vi "Matrix_Create.vi"(9 "Columns":i32, 11 "Rows":i32) -> (3 "output matrix":T1)   [LabVIEW 2019, in "Trajectory_Library.lvlib"]
doc: "Constructs an empty zero matrix of the given dimensions. \n\nInputs:\n - rows -- The number of rows of the matrix.\n - columns -- The number of columns of the matrix.\n\nOutputs:\n - output matrix -- Newly created matrix"
uses:
  Trajectory_Library.lvlib
  <vilib>/Analysis/Matrix/Datatypes/RealMatrix.ctl
  <vilib>/Analysis/Matrix/NI_Matrix.lvlib
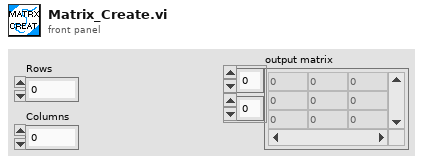
[diagram p1: front panel]
types:
  T1 = typedef "NI_Matrix.lvlib/RealMatrix.ctl" = dbl[][]
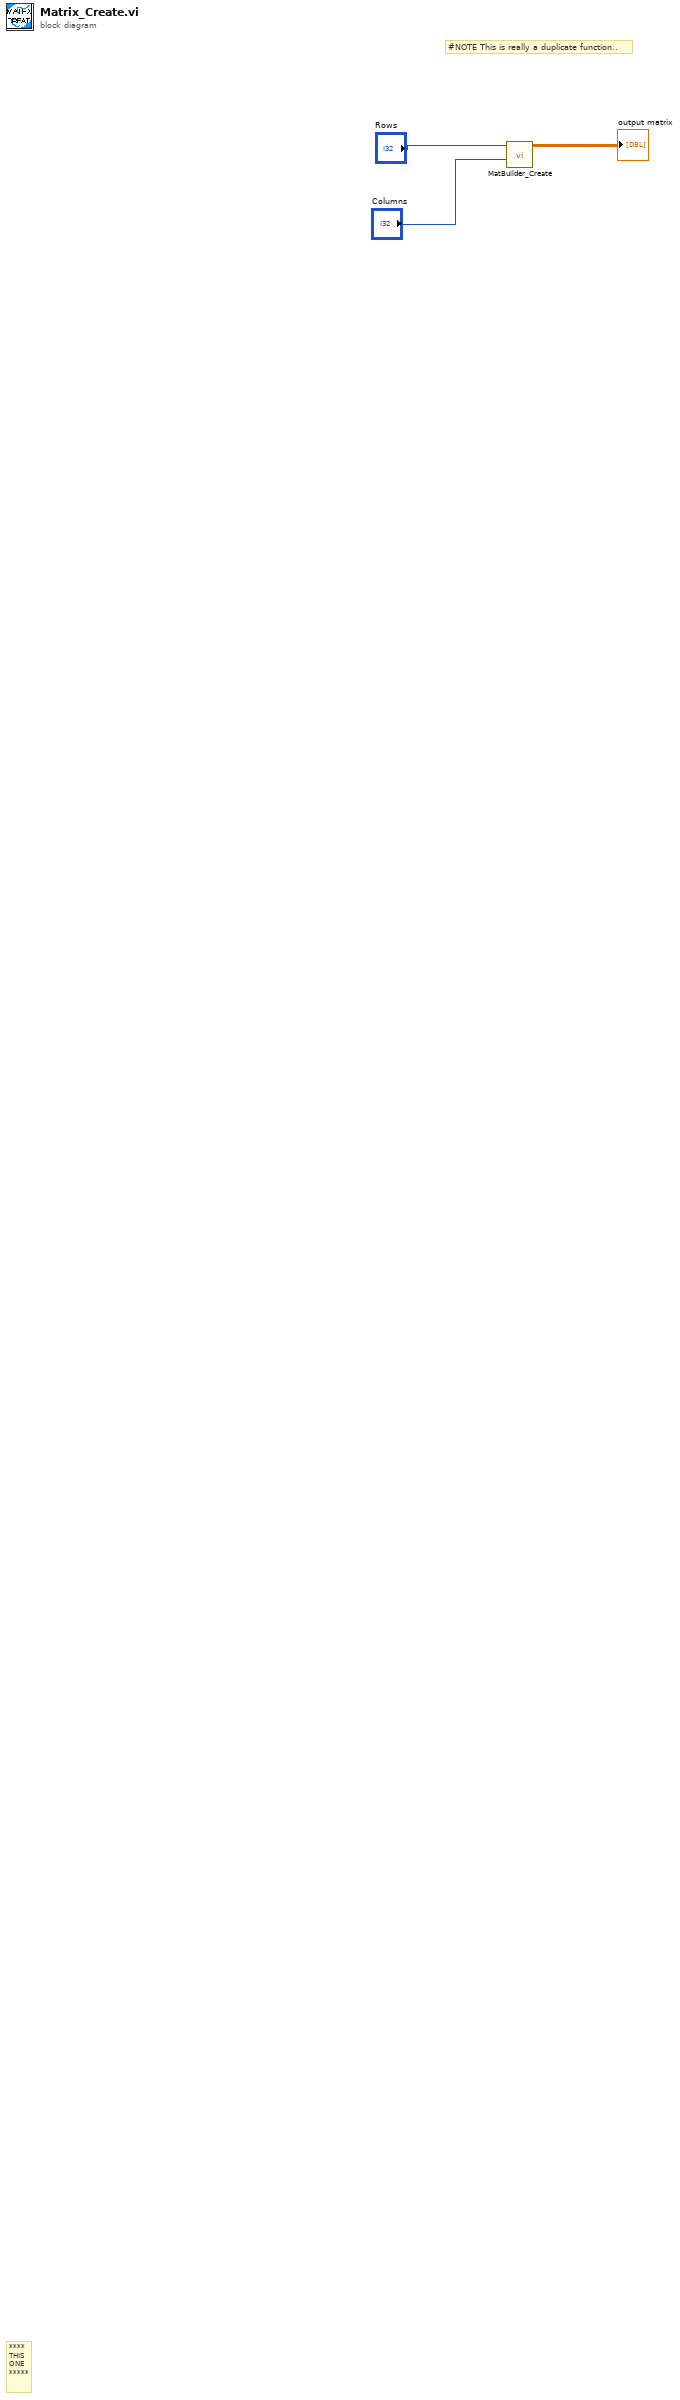
[diagram p0: block diagram]
diagram:
  # "#NOTE This is really a duplicate function.."
  # "****\nTHIS\nONE\n*****"
  n1 = call "MatBuilder_Create.vi"("Columns"="Columns", "Rows"="Rows") -> ("output matrix"=→"output matrix":T1)  [unwired: 9 in]
